vi "CreateDataSet.vi"(8 "error in (no error)":errorcluster, 9 "data":T10, 10 "data event":T2, 11 "config in":T1) -> (0 "error out":errorcluster, 2 "data event out":T2)   [LabVIEW 2017, in "IrDataEventCreator.lvlib"]
uses:
  <vilib>/addons/InsightCM/Devices/Shared/Ir/IrDataEventCreator/IrDataEventCreator.lvlib
  <vilib>/addons/InsightCM/Devices/Shared/Common/DataFlow/controls/Data.ctl
  <vilib>/addons/InsightCM/Utilities/DataAccessors/controls/wfmSGL_DVR.ctl
  <vilib>/addons/PointValueMap/controls/PointMap.ctl
  <vilib>/addons/InsightCM/Devices/Shared/Common/DataFlow/controls/Type.ctl
  <vilib>/addons/InsightCM/Devices/Shared/Common/DataEvent/controls/Event.ctl
  <vilib>/addons/InsightCM/MessageBus/Base/controls/DataEvent.ctl
  <vilib>/addons/InsightCM/MessageBus/Base/controls/KeyValuePair.ctl
  <vilib>/addons/InsightCM/Devices/Shared/Common/DataEvent/controls/DataSet.ctl
  <vilib>/addons/InsightCM/MessageBus/Base/controls/DataSetMetadata.ctl
  <vilib>/addons/InsightCM/MessageBus/Base/controls/TrendPoint.ctl
  <vilib>/addons/InsightCM/MessageBus/Base/controls/TrendAlarmUpdate.ctl
  <vilib>/addons/InsightCM/MessageBus/Base/controls/TrendAlarmTransition.ctl
  <vilib>/addons/InsightCM/Devices/Shared/Ir/IrDataEventCreator/controls/config.ctl
  <vilib>/addons/InsightCM/Devices/Shared/Common/DataEvent/controls/DataSetType.ctl
  <vilib>/addons/InsightCM/Devices/Shared/Ir/IrDataEventCreator/controls/Registry.ctl
  <vilib>/addons/InsightCM/Devices/Shared/Ir/IrDataEventCreator/controls/Registry_Image.ctl
  <vilib>/addons/InsightCM/Devices/Shared/Common/DataEventCreator/controls/Registry_Trend.ctl
  <vilib>/addons/InsightCM/Devices/Shared/Common/DataEvent/DataEvent.lvlib
  <vilib>/addons/InsightCM/SRP/SRP.lvlib
  <vilib>/addons/InsightCM/Utilities/PropertyHelpers/PropertyHelpers.lvlib
  <vilib>/addons/InsightCM/Devices/Shared/Common/DataEventCreator/DataEventCreator.lvlib
  <vilib>/addons/PointValueMap/PointValueMap.lvlib
  <vilib>/addons/InsightCM/Devices/Shared/Common/DataFlow/DataFlow.lvlib
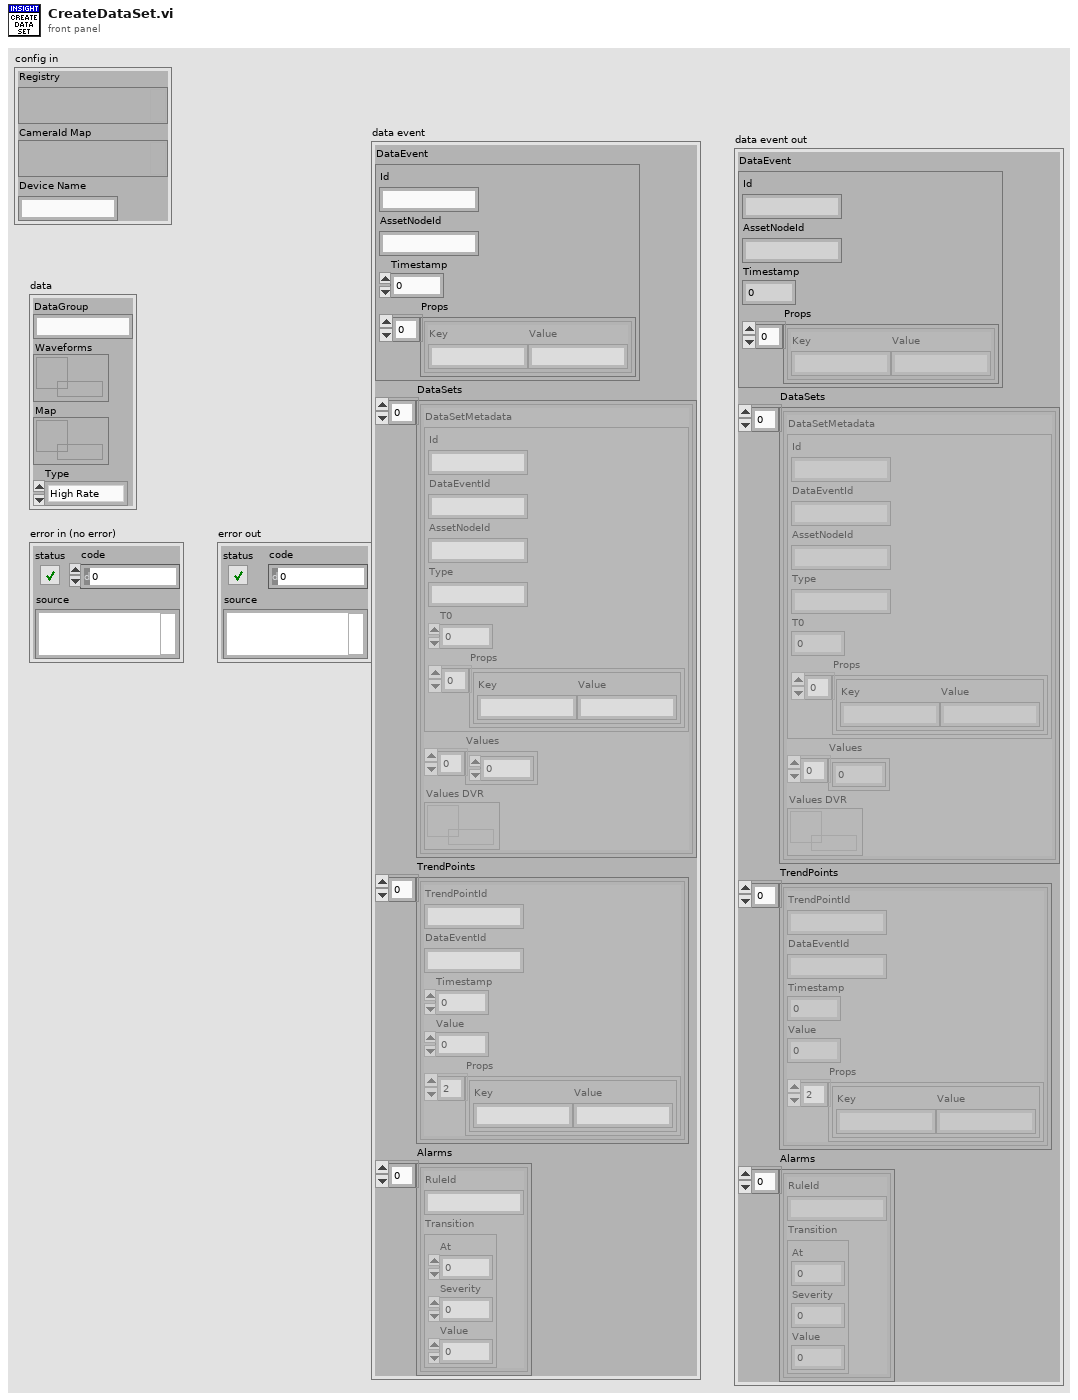
[diagram p1: front panel]
types:
  T1 = typedef "IrDataEventCreator.lvlib/config.ctl" = cluster{"Registry":variant, "CameraId Map":variant, "Device Name":string}
  T2 = typedef "DataEvent.lvlib/Event.ctl" = cluster{"DataEvent":T3, "DataSets":T5[], "TrendPoints":T7[], "Alarms":T8[]}
  T3 = typedef "DataEvent.ctl" = cluster{"Id":string, "AssetNodeId":string, "Timestamp":i64, "Props":T4[]}
  T4 = typedef "KeyValuePair.ctl" = cluster{"Key":string, "Value":string}
  T5 = typedef "DataEvent.lvlib/DataSet.ctl" = cluster{"DataSetMetadata":T6, "Values":sgl[], "Values DVR":refnum<data-value>}
  T6 = typedef "DataSetMetadata.ctl" = cluster{"Id":string, "DataEventId":string, "AssetNodeId":string, "Type":string, "T0":i64, "Props":T4[]}
  T7 = typedef "TrendPoint.ctl" = cluster{"TrendPointId":string, "DataEventId":string, "Timestamp":i64, "Value":dbl, "Props":T4[]}
  T8 = typedef "TrendAlarmUpdate.ctl" = cluster{"RuleId":string, "Transition":T9}
  T9 = typedef "TrendAlarmTransition.ctl" = cluster{"At":i64, "Severity":i32, "Value":dbl}
  T10 = typedef "DataFlow.lvlib/Data.ctl" = cluster{"DataGroup":string, "Waveforms":T11, "Map":T12, "Type":T13}
  T11 = typedef "wfmSGL_DVR.ctl" = refnum<data-value>
  T12 = typedef "PointValueMap.lvlib/PointMap.ctl" = refnum<data-value>
  T13 = typedef "DataFlow.lvlib/Type.ctl" = enum16{"High Rate", "Low Rate", "Burst Mode"}
  T14 = typedef "IrDataEventCreator.lvlib/Registry.ctl" = cluster{"Image":T15, "Trend Points":T16[]}
  T15 = typedef "IrDataEventCreator.lvlib/Registry_Image.ctl" = cluster{"Properties":T4[]}
  T16 = typedef "DataEventCreator.lvlib/Registry_Trend.ctl" = cluster{"TrendPointId":string, "DataSetName":string, "HighRate":bool, "Always Send":bool}
  T17 = typedef "DataEvent.lvlib/DataSetType.ctl" = enum16{"Waveform", "SpeedProfile", "ThermalImage", "EmsaSweep"}
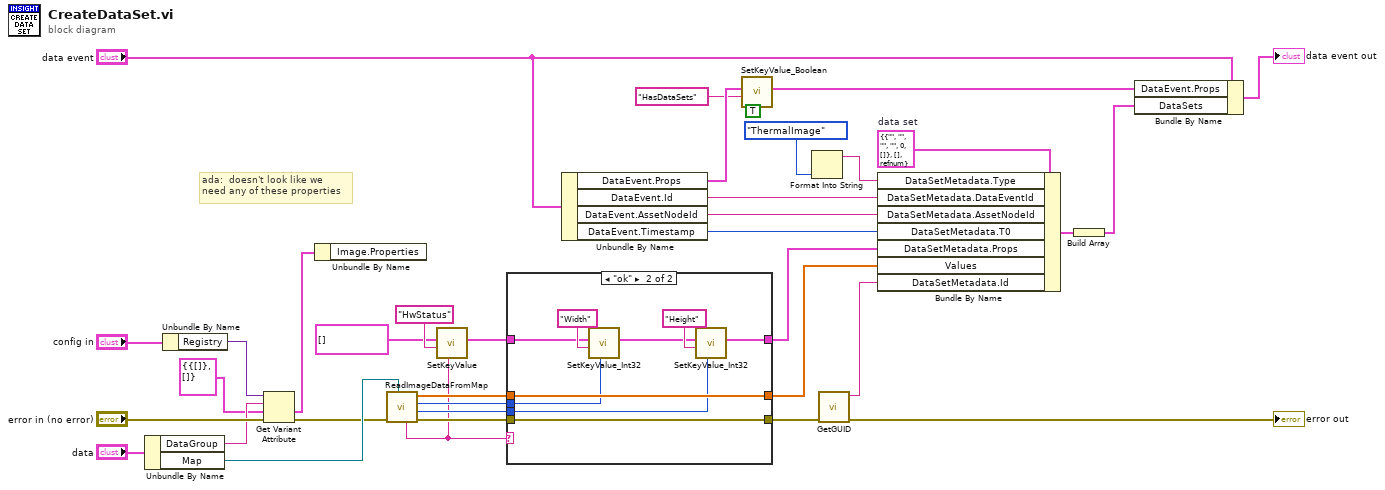
[diagram p0: block diagram]
diagram:
  w36 = T5 {"DataSetMetadata"={"Id"="", "DataEventId"="", "AssetNodeId"="", "Type"="", "T0"=0, "Props"=[]}, "Values"=[], "Values DVR"=refnum}  # data set
  # "ada:  doesn't look like we\nneed any of these properties"
  n1 = Unbundle By Name("data") -> ("DataGroup"=w20:string, "Map"=w7:T12)
  n2 = Unbundle By Name("config in") -> ("Registry"=w21:variant)
  n3 = Get Variant Attribute(Variant=w21, name=w20, default value (empty Variant)=T14 {"Image"={"Properties"=[]}, "Trend Points"=[]} ("Registry"), error in="error in (no error)") -> (value=w18:T14, error out=w6:errorcluster)  [unwired: 2 out]
  n4 = Unbundle By Name(w18) -> ()  [unwired: 1 out]
  n5 = call <vilib>:"ReadImageDataFromMap.vi"("map"=w7, "error in (no error)"=w6) -> ("error out"=w5:errorcluster, "image height"=w2:i32, "image width"=w3:i32, "image data"=w4:sgl[], "image status"=w1:string)  [unwired: 3 in, 2 out]
  n6 = call <vilib>:"SetKeyValue.vi"("value"=w1, "key"="HwStatus", "key value pairs"=T4[] []) -> ("key value pairs out"=w8:T4[])  [unwired: 8 in]
  n7 = case shown="\"ok\"" w1 {
    tunnel: w5 -> [w38 w42]
    tunnel: w8 -> [w37 w41]
    tunnel: [w37 w44] -> w25
    tunnel: [_ w43] -> w24
    tunnel: [w38 w42] -> w17
    tunnel: w4 -> [_ w43]
    tunnel: w3 -> [_ w40]
    tunnel: w2 -> [_ w39]
    frame Default {
    }
    frame "ok" {
      n8 = call <vilib>:"SetKeyValue_Int32.vi"("value"=w40, "key"="Width", "key value pairs"=w41) -> ("key value pairs out"=w45:T4[])  [unwired: 8 in]
      n9 = call <vilib>:"SetKeyValue_Int32.vi"("value"=w39, "key"="Height", "key value pairs"=w45) -> ("key value pairs out"=w44:T4[])  [unwired: 8 in]
    }
  }
  n10 = Unbundle By Name("data event") -> ("DataEvent.Props"=w12:T4[], "DataEvent.Id"=w33:string, "DataEvent.AssetNodeId"=w28:string, "DataEvent.Timestamp"=w26:i64)
  n11 = call <vilib>:"SetKeyValue_Boolean.vi"("value"=TRUE, "key"="HasDataSets", "key value pairs"=w12) -> ("key value pairs out"=w11:T4[])  [unwired: 8 in]
  n12 = Format Into String(DataSetType."ThermalImage" ("DataSetType")) -> (resulting string=w27:string)  [unwired: 3 in, 1 out]
  n13 = call <vilib>:"GetGUID.vi"("error in (no error)"=w17) -> ("error out"=→"error out":errorcluster, "GUID"=w15:string)  [unwired: 9 in]
  n14 = Bundle By Name(cluster=w36, "DataSetMetadata.Type"=w27, "DataSetMetadata.DataEventId"=w33, "DataSetMetadata.AssetNodeId"=w28, "DataSetMetadata.T0"=w26, "DataSetMetadata.Props"=w25, "Values"=w24, "DataSetMetadata.Id"=w15) -> (w32:T5)
  n15 = Build Array(w32) -> (w30:T5[])
  n16 = Bundle By Name(cluster="data event", "DataEvent.Props"=w11, "DataSets"=w30) -> (→"data event out":T2)
